vi "svmdense_predict.vi"(8 "error in (no error)":errorcluster, 10 "X":T1, 11 "Model":T2) -> (0 "error out":errorcluster, 3 "Predicted label":dbl)   [LabVIEW 2014]
doc: "This function does classification or regression on a test vector x given a model.\n\nFor a classification model, the predicted class for x is returned.\nFor a regression model, the function value of x calculated using the model is returned. For an one-class model, +1 or -1 is returned."
uses:
  Controls/svmdense_model.ctl
  LibSVM Sparse/Wrapper API/Controls/svm_parameter.ctl
  LibSVM Sparse/Wrapper API/Controls/svm_type.ctl
  LibSVM Sparse/Wrapper API/Controls/svm_kernel_type.ctl
  Controls/svmdense_node.ctl
  bin/x64/LabVIEW-libsvm-dense.dll
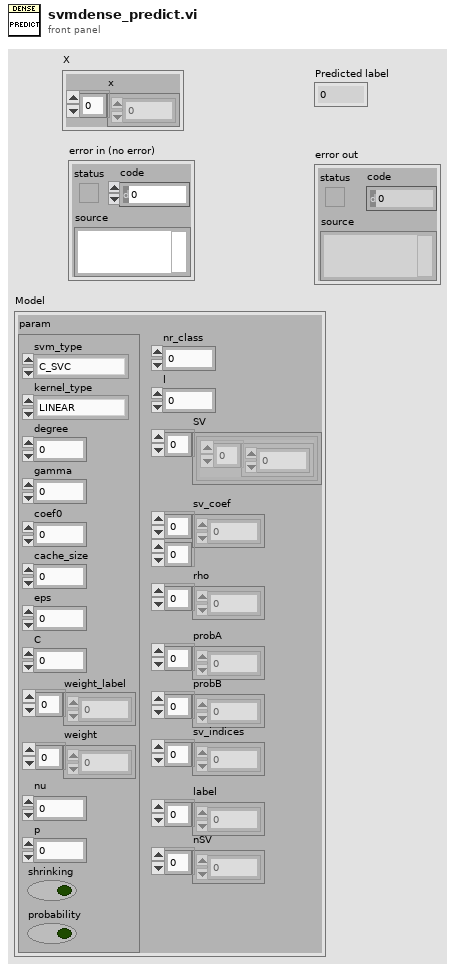
[diagram p1: front panel]
types:
  T1 = typedef "svmdense_node.ctl" = cluster{"x":dbl[]}
  T2 = typedef "svmdense_model.ctl" = cluster{"param":T3, "nr_class":i32, "l":i32, "SV":cluster{"Array":dbl[]}[], "sv_coef":dbl[][], "rho":dbl[], "probA":dbl[], "probB":dbl[], "sv_indices":i32[], "label":i32[], "nSV":i32[]}
  T3 = typedef "svm_parameter.ctl" = cluster{"svm_type":T4, "kernel_type":T5, "degree":i32, "gamma":dbl, "coef0":dbl, "cache_size":dbl, "eps":dbl, "C":dbl, "weight_label":i32[], "weight":dbl[], "nu":dbl, "p":dbl, "shrinking":bool, "probability":bool}
  T4 = typedef "svm_type.ctl" = enum32{"C_SVC", "NU_SVC", "ONE_CLASS", "EPSILON_SVR", "NU_SVR"}
  T5 = typedef "svm_kernel_type.ctl" = enum32{"LINEAR", "POLY", "RBF", "SIGMOID", "PRECOMPUTED"}
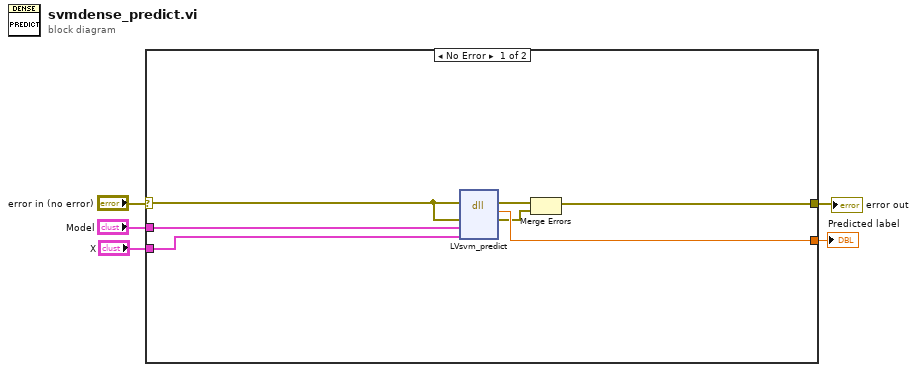
[diagram p0: block diagram]
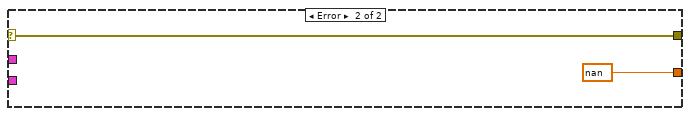
[diagram p2: hidden frame]
diagram:
  n1 = case shown="No Error" "error in (no error)" {
    selector: "error in (no error)" -> [w12 w14]
    tunnel: [w11 w14] -> w5
    tunnel: "Model" -> [w10 _]
    tunnel: "X" -> [w9 _]
    tunnel: [w8 nan ("predicted label")] -> w3
    frame No Error {
      n2 = dll-call lib="C:/dev/LabVIEW-libsvm/LabVIEW/bin/x64/LabVIEW-libsvm-dense.dll" fn="LVsvm_predict"(error in=w12, "lvErr"=w12, "model_in"=w10, "x_in"=w9) -> (error out=w7:errorcluster, "predicted label"=w8:dbl, "lvErr"=w6:errorcluster)  [unwired: 4 in, 1 out]
      n3 = Merge Errors(w7, w6) -> (w11:errorcluster)
    }
    frame Error {
    }
  }
  "error out" <- w5
  "Predicted label" <- w3
